vi "PH_ImageOperator.PC set Global On.vi"(0 "i ref in":refnum<vi>, 2 "Global On":bool, 5 "error in (no error)":errorcluster) -> (14 "i ref out":refnum<vi>, 19 "error out":errorcluster)   [LabVIEW 2014, in "PH_ImageOperator.lvlib"]
doc: "This VI switches the periodic loop on or off and sets some GUI elements."
uses:
  PH_ImageOperator.lvlib
  CS_Core/BaseProcess/BaseProcess.lvlib
  PH_Basics/PH_Common/PH_Common.lvlib
  PH_Basics/PH_Img_BaseClass/PH_Img_BaseClass.lvlib
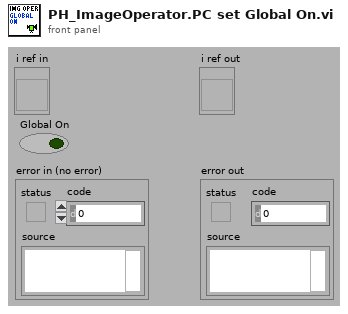
[diagram p1: front panel]
types:
  T1 = typedef "PH_Img_BaseClass.lvlib/PH_Img_BaseClass.i attribute.ctl" = cluster{"GUI Refs":T2, "Timeout Image [ms]":i32, "Default Periodic Period [ms]":i32, "Camera":cluster{"Instancename":string, "Notifier":refnum<notifier>}, "Palette":T3, "Cam Settings":cluster{"Cam ID":string, "Gain":dbl, "Brightness":dbl, "Shutter":dbl, "Cam Info Failure":bool, "Mode":i32}}
  T2 = typedef "PH_Img_BaseClass.lvlib/PH_Img_BaseClass.GUI Refs.ctl" = cluster{"Timeout":refnum<vi>, "Image":refnum<vi>, "Palette":refnum<vi>, "Timeout Set":refnum<vi>}
  T3 = typedef "PH_Img_BaseClass.lvlib/PH_Img_BaseClass.Palette.ctl" = i32
  T4 = typedef "PH_ImageOperator.lvlib/PH_ImageOperator.i attribute.ctl" = cluster{"GUI Refs":cluster{"Delete":refnum<vi>, "Calibration status":refnum<vi>, "BI subtracted":refnum<vi>, "calc Energy":refnum<vi>, "Energy: expected value":refnum<vi>, "Energy: Tolerance":refnum<vi>, "Energy calculated":refnum<vi>, "Energy":refnum<vi>, "calc Beam Anal":refnum<vi>, "Maj Diam 1/esquare":refnum<vi>, "Min Diam 1/esquare":refnum<vi>, "Azi Angle":refnum<vi>, "Min/Maj Diam esquare":refnum<vi>, "Beam analysed":refnum<vi>, "CoG - x":refnum<vi>, "CoG - y":refnum<vi>, "BA: Method":refnum<vi>, "BA: Steps":refnum<vi>, "BA: Factor":refnum<vi>, "calc Traces":refnum<vi>, "Traces: Fit Gauss":refnum<vi>, "Traces calculated":refnum<vi>, "Maj FWHM":refnum<vi>, "Min FWHM":refnum<vi>, "Major Trace":refnum<vi>, "Minor Trace":refnum<vi>, "Maj Fit Order":refnum<vi>, "Min Fit Order":refnum<vi>, "Position calculated":refnum<vi>, "Position":refnum<vi>, "Type":refnum<vi>, "Center":refnum<vi>, "exp - X":refnum<vi>, "exp - Y":refnum<vi>, "Tolerance":refnum<vi>, "f":refnum<vi>, "M":refnum<vi>, "D":refnum<vi>, "q":refnum<vi>, "Dummy Method":refnum<vi>, "Dummy Type":refnum<vi>, "Global On":refnum<vi>, "Traces: No offset":refnum<vi>, "Maj 99%":refnum<vi>, "Min 99%":refnum<vi>, "GUI FF Image":refnum<vi>, "calc Fill Factor":refnum<vi>, "FF calculated":refnum<vi>, "Fill Factor: Filter?":refnum<vi>, "FF: Damage Threshold":refnum<vi>, "FF: Threshold":refnum<vi>, "FF: max allow. Energy":refnum<vi>, "FF: Fillfactor":refnum<vi>, "Calibration data":refnum<vi>}, "List of GUIs":string[], "Calibration":cluster{"Status":T5, "Calibration data":T6, "Calibration Data File":path}, "Final Image":cluster{"BI Subtraction Failure":bool}, "Energy":cluster{"on":bool, "expected value [mJ]":dbl, "Tolerance [%]":dbl, "State":T5, "Energy [mJ]":dbl, "Unit":string, "calculated @":timestamp}, "Beam Analysis":cluster{"on":bool, "Data":T7, "Method":bool, "Steps":i32, "Factor":i32, "ROI":cluster{"Left":i32, "Top":i32, "Right":i32, "Bottom":i32}, "analysed @":timestamp}, "Trace Analysis":cluster{"on":bool, "Fit on":bool, "Maj FWHM":dbl, "Min FWHM":dbl, "Maj Fit Order":i32, "Min Fit Order":i32, "No Offset":bool, "Maj 99%":dbl, "Min 99%":dbl, "Traces":cluster{"XScaleName":string, "Y Scale Minimum":sgl, "Y Scale Maximum":sgl, "X Scale Minimum":sgl, "X Scale Maximum":sgl, "Traces":cluster{"Index":sgl[], "Trace":dbl[]}[]}[], "analysed @":timestamp}, "Position Analysis":cluster{"on":bool, "exp - X":i32, "exp - Y":i32, "focal length [mm]":dbl, "Magnification":dbl, "Delta":dbl, "Theta":dbl, "Tolerance":dbl, "Type":bool, "analysed @":timestamp}, "Fill Factor":cluster{"on":bool, "Filter on?":bool, "Threshold":dbl, "Damage Threshold [J/cm²]":dbl, "Fillfactor":dbl, "Max. allowed Energy [J]":dbl, "calculated @":timestamp}, "Statistician Service ID":i32, "Images":cluster{"Background":T8, "OP":T8, "GUI":T8, "BA: ROI":T8, "Trace: Turn":T8, "FF: Main":T8, "FF: Help":T8, "PSDB: BG":T8, "PSDB: OP":T8, "PSDB: FF":T8}}
  T5 = typedef "PH_StatusHandler.lvlib/PH_StatusHandler.Status.ctl" = i16
  T6 = typedef "PH_ImageCalibrator.lvlib/PH_ImageCalibrator.Calibration Data.ctl" = cluster{"Date":string, "Time":string, "Cam Settings":cluster{"Cam ID":string, "Gain":dbl, "Brightness":dbl, "Shutter":dbl, "Cam Error":bool, "Mode":i32}, "Background Image":cluster{"Image":dbl[][], "Image Error":bool}, "Linear Calibration":cluster{"Calibration Factor":dbl, "not mm or mrad":bool}, "Energy Calibration":cluster{"Calibration Factor":dbl, "no mJ":bool}}
  T7 = typedef "PH_ImageOperator.lvlib/PH_ImageOperator.Beam Analysis Data.ctl" = cluster{"CoG-x":sgl, "CoG-y":sgl, "Maj Dim":dbl, "Min Dim":dbl, "Ellipticity":dbl, "Azimuth Angle [rad]":dbl, "Azi Angle rel to Maj?":bool}
  T8 = typedef "IMAQ Image.ctl" = refnum<image>
  T9 = enum16{"simple", "synchronous", "asynchronous", "notification"}
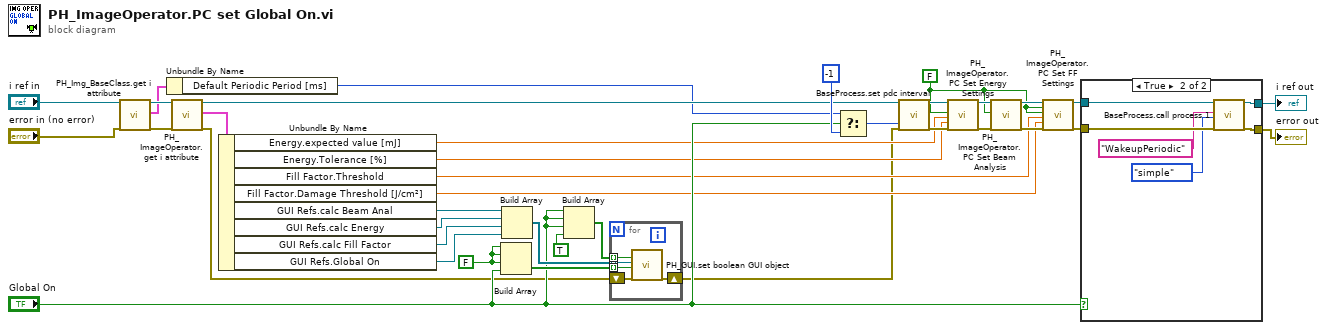
[diagram p0: block diagram]
diagram:
  w10 = FALSE ("Calc Energy")
  w24 = FALSE ("element")
  n1 = call "PH_Img_BaseClass.get i attribute.vi"("i ref in"="i ref in", "error in (no error)"="error in (no error)") -> ("i ref out"=w6:refnum<vi>, "i attribute"=w3:T1, "error out"=w5:errorcluster)  [unwired: 15 in]
  n2 = Unbundle By Name(w3) -> ("Default Periodic Period [ms]"=w2:i32)
  n3 = call "PH_ImageOperator.get i attribute.vi"("i ref in"=w6, "error in (no error)"=w5) -> ("i ref out"=w28:refnum<vi>, "i attribute"=w37:T4, "error out"=w9:errorcluster)  [unwired: 15 in]
  n4 = Unbundle By Name(w37) -> ("Energy.expected value [mJ]"=w18:dbl, "Energy.Tolerance [%]"=w17:dbl, "Fill Factor.Threshold"=w8:dbl, "Fill Factor.Damage Threshold [J/cm²]"=w7:dbl, "GUI Refs.calc Beam Anal"=w36:refnum<vi>, "GUI Refs.calc Energy"=w35:refnum<vi>, "GUI Refs.calc Fill Factor"=w34:refnum<vi>, "GUI Refs.Global On"=w27:refnum<vi>)
  n5 = Build Array(w24, w24, w24, "Global On") -> (w25:bool[])
  n6 = Build Array(w36, w35, w34, w27) -> (w26:refnum<vi>[])
  n7 = Build Array("Global On", "Global On", "Global On", TRUE ("element")) -> (w21:bool[])
  n8 = for {
    shift-right: [w41] -> w1
    shift-left: w9 -> [w42]
    tunnel: w26 -> [w40] mode=indexing
    tunnel: w25 -> [w39] mode=indexing
    tunnel: w21 -> [w38] mode=indexing
    n9 = call "PH_GUI.set boolean GUI object.vi"("Visible (true)"=w38, "Boolean Knob GUI Ref"=w40, "Value"=w39, "error in (no error)"=w42) -> ("error out"=w41:errorcluster)  [unwired: 15 in]
  }
  n10 = Select(t=w2, s="Global On", f=-1 ("PeriodicInterval")) -> (s? t:f=w31:i32)
  n11 = call "BaseProcess.set pdc interval.vi"("i ref in"=w28, "PeriodicInterval [ms]"=w31, "error in (no error)"=w1) -> ("i ref out"=w20:refnum<vi>, "error out"=w19:errorcluster)  [unwired: 14 in, 1 out]
  n12 = call "PH_ImageOperator.PC Set Energy Settings.vi"("i ref in"=w20, "Calc Energy"=w10, "Expected Value [mJ]"=w18, "Tolerance [%]"=w17, "error in (no error)"=w19) -> ("i ref out"=w16:refnum<vi>, "error out"=w15:errorcluster)  [unwired: 13 in]
  n13 = call "PH_ImageOperator.PC Set Beam Analysis.vi"("i ref in"=w16, "On / Off"=w10, "error in"=w15) -> ("i ref out"=w12:refnum<vi>, "error out"=w14:errorcluster)  [unwired: 15 in]
  n14 = call "PH_ImageOperator.PC Set FF Settings.vi"("i ref in"=w12, "Calc Fill Factor"=w10, "Filter"=w10, "Threshold"=w8, "Damage Threshold [J/cm²]"=w7, "error in (no error)"=w14) -> ("i ref out"=w11:refnum<vi>, "error out"=w13:errorcluster)  [unwired: 12 in]
  n15 = case shown="True" "Global On" {
    tunnel: [w44 w50] -> w30
    tunnel: w13 -> [w43 w49]
    tunnel: [w43 w48] -> w29
    tunnel: w11 -> [w44 w47]
    frame False {
    }
    frame True {
      n16 = call "BaseProcess.call process 1.vi"("i ref in"=w47, "Selector"="WakeupPeriodic", "CallType"=T9."simple", "error in (no error)"=w49) -> ("i ref out"=w50:refnum<vi>, "error out"=w48:errorcluster)  [unwired: 13 in, 1 out]
    }
  }
  "error out" <- w29
  "i ref out" <- w30
